vi "CH_LM App FGV DCLRefs.vi"(7 "Function":T1=enum."get", 8 "error in (no error)":errorcluster, 9 "VI Name":string, 11 "VI Ref":refnum<vi>) -> (0 "error out":errorcluster, 1 "VI Name":string, 3 "VI Ref":refnum<vi>, 4 "VI Names":string[](array[string]), 5 "VI Refs":refnum<vi>[](array[refnum]), 6 "empty":bool)   [LabVIEW 2012, in "CH_LM App.lvlib"]
doc: "This functional global variable maintains the VI Refs of all LabMax DAQ threads."
uses:
  CH_LM App.lvlib
  CH_LM.lvlib
  _CH_LM/CH_LM FGV Functions.ctl
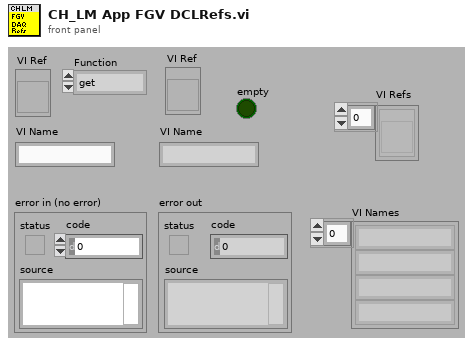
[diagram p1: front panel]
types:
  T1 = typedef "CH_LM.lvlib/CH_LM FGV Functions.ctl" = enum16{"create", "get", "set", "remove", "clear", "getBySerial"}
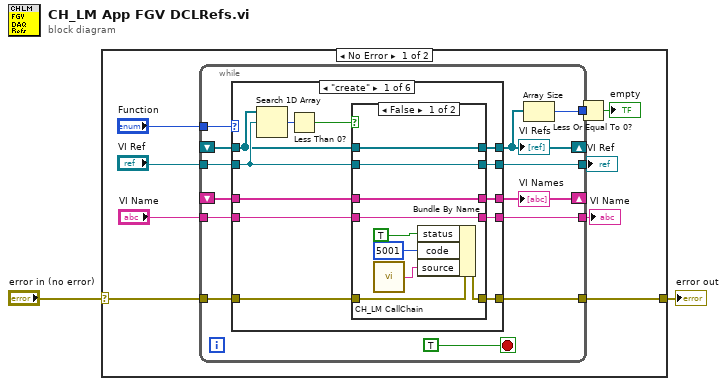
[diagram p0: block diagram]
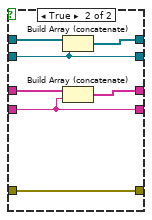
[diagram p2: hidden frame]
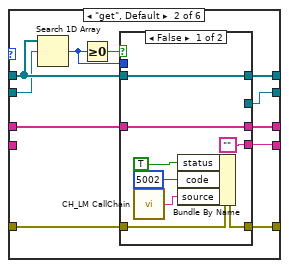
[diagram p3: hidden frame]
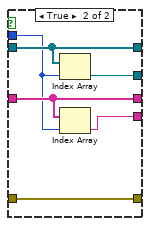
[diagram p4: hidden frame]
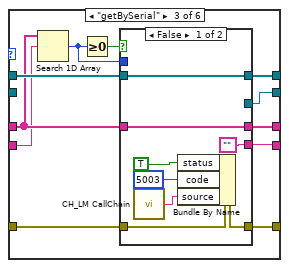
[diagram p5: hidden frame]
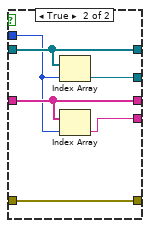
[diagram p6: hidden frame]
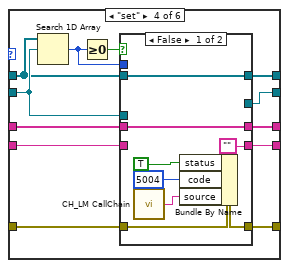
[diagram p7: hidden frame]
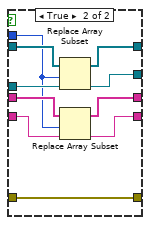
[diagram p8: hidden frame]
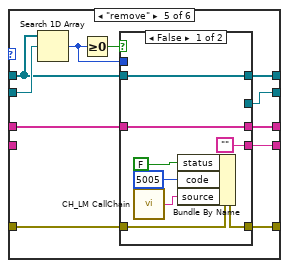
[diagram p9: hidden frame]
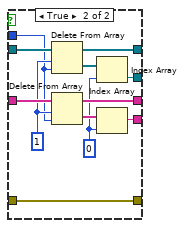
[diagram p10: hidden frame]
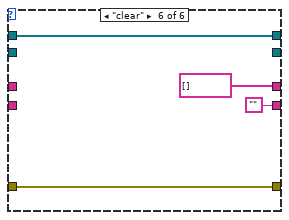
[diagram p11: hidden frame]
diagram:
  n1 = case shown="No Error" "error in (no error)" {
    selector: "error in (no error)" -> [w10 w166]
    tunnel: [w9 w166] -> w1
    frame No Error {
      n2 = while {
        tunnel: "Function" -> [w23]
        shift-right: [w12] -> _
        shift-left: _ -> [w21]
        tunnel: "VI Ref" -> [w22]
        tunnel: [w20] -> w5
        tunnel: w10 -> [w19]
        tunnel: [w18] -> w9
        shift-right: [w16] -> _
        shift-left: _ -> [w15]
        tunnel: "VI Name" -> [w17]
        tunnel: [w14] -> w7
        tunnel: [w13] -> w4
        stop <- TRUE stop-if-true
        n3 = case shown="\"create\"" w23 {
          tunnel: w22 -> [w27 w53 _ w104 w132 _]
          tunnel: w21 -> [w26 w54 w88 w103 w131 w162]
          tunnel: [w36 w59 w83 w109 w136 w162] -> w12
          tunnel: [w34 w58 w82 w114 w141 _] -> w20
          tunnel: w19 -> [w33 w61 w85 w111 w138 w165]
          tunnel: [w32 w60 w84 w110 w137 w165] -> w18
          tunnel: w17 -> [w31 _ w78 w106 _ _]
          tunnel: [w30 w56 w81 w107 w134 string[] []] -> w16
          tunnel: w15 -> [w29 w57 w79 w108 w135 _]
          tunnel: [w28 w55 w80 w105 w133 ""] -> w14
          frame "create" {
            n4 = Search 1D Array(1D array=w26, element=w27) -> (index of element=w35:i32)  [unwired: 1 out]
            n5 = Less Than 0?(x=w35) -> (x < 0?=w25:bool)
            n6 = case shown="False" w25 {
              tunnel: w27 -> [w44 w50]
              tunnel: w26 -> [w45 w52]
              tunnel: [w45 w51] -> w36
              tunnel: [w44 w50] -> w34
              tunnel: w33 -> [w43 w49]
              tunnel: [w42 w49] -> w32
              tunnel: w31 -> [w37 w46]
              tunnel: [w38 w48] -> w30
              tunnel: w29 -> [w38 w47]
              tunnel: [w37 w46] -> w28
              frame False {
                n7 = call "CH_LM CallChain.vi"() -> ("ChallChain"=w39:string)
                n8 = Bundle By Name(cluster=w43, "status"=TRUE, "code"=5001, "source"=w39) -> (w42:errorcluster)
              }
              frame True {
                n9 = Build Array (concatenate)(w52, w50) -> (w51:refnum<vi>[])
                n10 = Build Array (concatenate)(w47, w46) -> (w48:string[])
              }
            }
          }
          frame "get", Default {
            n11 = Search 1D Array(1D array=w54, element=w53) -> (index of element=w63:i32)  [unwired: 1 out]
            n12 = Greater Or Equal To 0?(x=w63) -> (x >= 0?=w62:bool)
            n13 = case shown="False" w62 {
              tunnel: w54 -> [w66 w75]
              tunnel: [_ w77] -> w58
              tunnel: w63 -> [_ w72]
              tunnel: w61 -> [w68 w76]
              tunnel: [w67 w76] -> w60
              tunnel: [w66 w75] -> w59
              tunnel: w57 -> [w65 w74]
              tunnel: [w65 w74] -> w56
              tunnel: ["" w73] -> w55
              frame False {
                n14 = call "CH_LM CallChain.vi"() -> ("ChallChain"=w69:string)
                n15 = Bundle By Name(cluster=w68, "status"=TRUE, "code"=5002, "source"=w69) -> (w67:errorcluster)
              }
              frame True {
                n16 = Index Array(array=w75, index=w72) -> (element=w77:refnum<vi>)
                n17 = Index Array(array=w74, index=w72) -> (element=w73:string)
              }
            }
          }
          frame "getBySerial" {
            n18 = Search 1D Array(1D array=w79, element=w78) -> (index of element=w87:i32)  [unwired: 1 out]
            n19 = Greater Or Equal To 0?(x=w87) -> (x >= 0?=w86:bool)
            n20 = case shown="False" w86 {
              tunnel: w88 -> [w91 w100]
              tunnel: [_ w102] -> w82
              tunnel: w87 -> [_ w97]
              tunnel: w85 -> [w93 w101]
              tunnel: [w92 w101] -> w84
              tunnel: [w91 w100] -> w83
              tunnel: w79 -> [w90 w99]
              tunnel: [w90 w99] -> w81
              tunnel: ["" w98] -> w80
              frame False {
                n21 = call "CH_LM CallChain.vi"() -> ("ChallChain"=w94:string)
                n22 = Bundle By Name(cluster=w93, "status"=TRUE, "code"=5003, "source"=w94) -> (w92:errorcluster)
              }
              frame True {
                n23 = Index Array(array=w100, index=w97) -> (element=w102:refnum<vi>)
                n24 = Index Array(array=w99, index=w97) -> (element=w98:string)
              }
            }
          }
          frame "set" {
            n25 = Search 1D Array(1D array=w103, element=w104) -> (index of element=w113:i32)  [unwired: 1 out]
            n26 = Greater Or Equal To 0?(x=w113) -> (x >= 0?=w112:bool)
            n27 = case shown="False" w112 {
              tunnel: w103 -> [w117 w128]
              tunnel: [_ w129] -> w114
              tunnel: w113 -> [_ w123]
              tunnel: w111 -> [w119 w130]
              tunnel: [w118 w130] -> w110
              tunnel: [w117 w127] -> w109
              tunnel: w104 -> [_ w129]
              tunnel: w108 -> [w116 w126]
              tunnel: [w116 w125] -> w107
              tunnel: w106 -> [_ w124]
              tunnel: ["" w124] -> w105
              frame False {
                n28 = call "CH_LM CallChain.vi"() -> ("ChallChain"=w120:string)
                n29 = Bundle By Name(cluster=w119, "status"=TRUE, "code"=5004, "source"=w120) -> (w118:errorcluster)
              }
              frame True {
                n30 = Replace Array Subset(array=w128, new element=w129, index=w123) -> (w127:refnum<vi>[])
                n31 = Replace Array Subset(array=w126, new element=w124, index=w123) -> (w125:string[])
              }
            }
          }
          frame "remove" {
            n32 = Search 1D Array(1D array=w131, element=w132) -> (index of element=w140:i32)  [unwired: 1 out]
            n33 = Greater Or Equal To 0?(x=w140) -> (x >= 0?=w139:bool)
            n34 = case shown="False" w139 {
              tunnel: w131 -> [w144 w160]
              tunnel: [_ w158] -> w141
              tunnel: w140 -> [_ w151]
              tunnel: w138 -> [w146 w161]
              tunnel: [w145 w161] -> w137
              tunnel: [w144 w159] -> w136
              tunnel: w135 -> [w143 w155]
              tunnel: [w143 w154] -> w134
              tunnel: ["" w153] -> w133
              frame False {
                n35 = call "CH_LM CallChain.vi"() -> ("ChallChain"=w147:string)
                n36 = Bundle By Name(cluster=w146, "status"=FALSE, "code"=5005, "source"=w147) -> (w145:errorcluster)
              }
              frame True {
                w150 = 0 ("index")
                w152 = 1 ("length")
                n37 = Delete From Array(array=w160, length=w152, index=w151) -> (deleted portion=w157:refnum<vi>[], array with subset deleted=w159:refnum<vi>[])
                n38 = Delete From Array(array=w155, length=w152, index=w151) -> (deleted portion=w156:string[], array with subset deleted=w154:string[])
                n39 = Index Array(array=w157, index=w150) -> (element=w158:refnum<vi>)
                n40 = Index Array(array=w156, index=w150) -> (element=w153:string)
              }
            }
          }
          frame "clear" {
          }
        }
        "VI Names" <- w16
        "VI Refs" <- w12
        n41 = Array Size(array=w12) -> (size(s)=w13:i32)
      }
      "VI Name" <- w7
      "VI Ref" <- w5
      n42 = Less Or Equal To 0?(x=w4) -> (x <= 0?=→"empty":bool)
    }
    frame Error {
    }
  }
  "error out" <- w1
